vi "Fetch.vi"(8 "error in (no error)":errorcluster, 10 "Message in":refnum<class "FetchMessage.lvclass">, 11 "MeritFactor in":refnum<class "MeritFactor.lvclass">) -> (0 "error out":errorcluster, 3 "MeritFactor out":refnum<class "MeritFactor.lvclass">)   [LabVIEW 2012, in "MeritFactor.lvclass"]
doc: "The fetch method processes the command 'fetch'. \n\nThe command 'fetch' is used for receiving various forms of data."
uses:
  MeritFactor.lvclass
  <vilib>/Distrio/Murmex/FetchMessage/FetchMessage.lvclass
  <vilib>/Distrio/Murmex/Murmex/Murmex.lvclass
  MeritFactor.lvclass/MeritFactor.ctl
  <vilib>/vision/Image Controls.llb/IMAQ Image.ctl
  <vilib>/vision/NI_Vision_Development_Module.lvlib
panel:
  out "Histogram Report":T1 {"Standard  Variation" format="%.2f"; "Mean Value" format="%.2f"; "Interval Width" format="%.2f"; "Starting Value" format="%.2f"; "Maximal Value" format="%.2f"; "Minimal Value" format="%.2f"}
  # "This method is called when the FETCH\ntrigger is sent. \n\nOverride this method when your component needs to\nrespond to this trigger. \n\nCall parent for proper implementation"
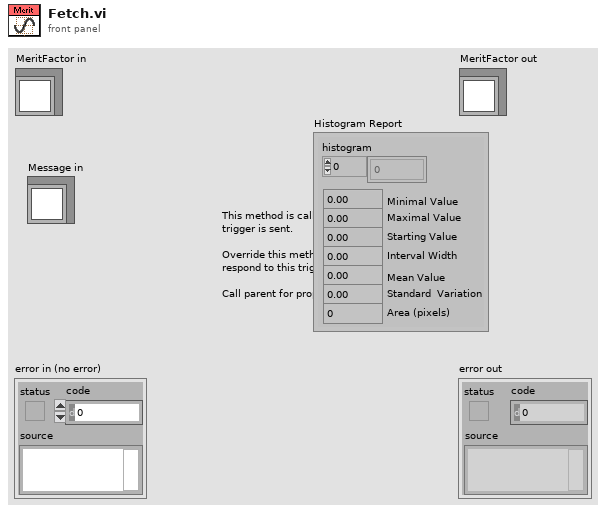
[diagram p1: front panel]
types:
  T1 = cluster{"histogram":u32[], "Minimal Value":sgl, "Maximal Value":sgl, "Starting Value":sgl, "Interval Width":sgl, "Mean Value":sgl, "Standard  Variation":sgl, "Area (pixels)":i32}
  T2 = typedef "IMAQ Image.ctl" = refnum<image>
  T3 = typedef "Murmex.lvlib/FetchMessage.lvclass/Channel data cluster.ctl" = cluster{"channel id":i32, "data UInt8":u8[], "data type":T4, "dimensions":i32[], "physical units":T5[], "waveform dt":dbl, "waveform":T6}
  T4 = typedef "Murmex.lvlib/Murmex.lvclass/data_type_enum.ctl" = enum16{"Float128", "Float64", "Float32", "Int64", "Int32", "Int16", "Int8", "UInt64", "UInt32", "UInt16", "UInt8", "Boolean", "String"}
  T5 = typedef "Physical Units__ogtk.ctl" = cluster{"Base Units":enum16{"radian", "steradian", "second", "meter", "kilogram", "ampere", "kelvin", "mole", "candela"}, "Exponent":i16}
  T6 = typedef "Murmex.lvlib/Murmex.lvclass/waveform_type_enum.ctl" = enum16{"no waveform", "analog", "digital"}
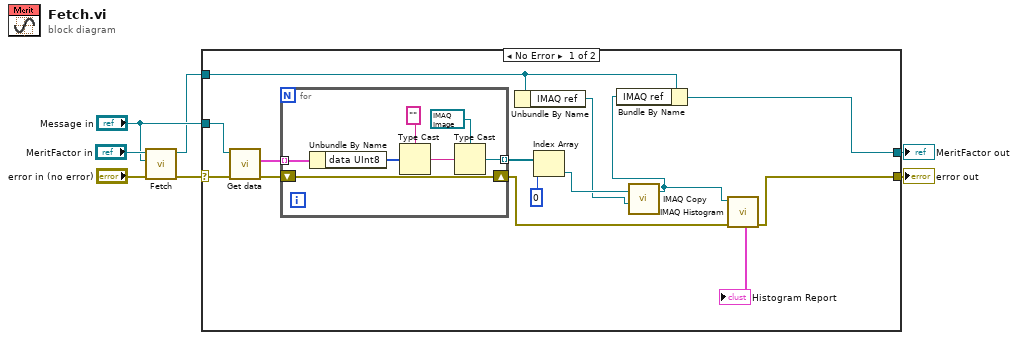
[diagram p0: block diagram]
diagram:
  n1 = call-parent "Fetch.vi"("error in (no error)"="error in (no error)", "Message in"="Message in", "Murmex in"="MeritFactor in") -> ("error out"=w5:errorcluster, "Murmex out"=w3:refnum<class "MeritFactor.lvclass">)  [unwired: 7 in]
  n2 = case shown="No Error" w5 {
    selector: w5 -> [w21 w29]
    tunnel: "Message in" -> [w18 _]
    tunnel: w3 -> [w11 w30]
    tunnel: [w13 w30] -> w2
    tunnel: [w14 w29] -> w1
    frame No Error {
      n3 = call <vilib>:"Get data.vi"("error in (no error)"=w21, "FetchMessage.lvclass"=w18) -> ("error out"=w20:errorcluster, "data (channels)"=w19:T3[])  [unwired: 7 in, 1 out]
      n4 = for {
        shift-right: [w27] -> w15
        shift-left: w20 -> [w27]
        tunnel: w19 -> [w28] mode=indexing
        tunnel: [w24] -> w17 mode=indexing
        n5 = Unbundle By Name(w28) -> ("data UInt8"=w26:u8[])
        n6 = Type Cast(type="", x=w26) -> (*(type *) &x=w23:string)
        n7 = Type Cast(type=T2 refnum ("Image"), x=w23) -> (*(type *) &x=w24:T2)
      }
      n8 = Unbundle By Name(w11) -> ("IMAQ ref"=w8:T2)
      n9 = Index Array(array=w17, index=0 ("index (row)")) -> (element=w9:T2)
      n10 = call "IMAQ Copy"("Image Dst"=w8, "Image Src"=w9) -> ("Image Dst Out"=w10:T2)  [unwired: 4 in, 1 out]
      n11 = Bundle By Name(cluster=w11, "IMAQ ref"=w10) -> (w13:refnum<class "MeritFactor.lvclass">)
      n12 = call "IMAQ Histogram"("error in (no error)"=w15, "Image"=w10) -> ("error out"=w14:errorcluster, "Histogram Report"=→"Histogram Report":T1)  [unwired: 8 in]
    }
    frame Error {
    }
  }
  "error out" <- w1
  "MeritFactor out" <- w2
